vi "_get Session Name for PN.vi"(8 "error in (no error)":errorcluster, 11 "OBJ - Session in":refnum<class "Session - Root.lvclass">) -> (0 "error out":errorcluster, 2 "Session Name":string, 3 "OBJ - Session out":refnum<class "Session - Root.lvclass">)   [LabVIEW 2015, in "Session - Root.lvclass"]
doc: "Wrapped Call to maintain reverse compatibility\nOnly difference is connector pane"
uses:
  Session - Root.lvclass
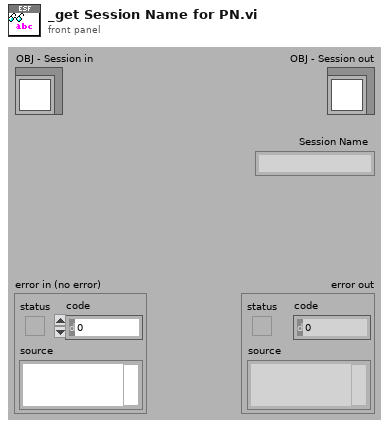
[diagram p1: front panel]
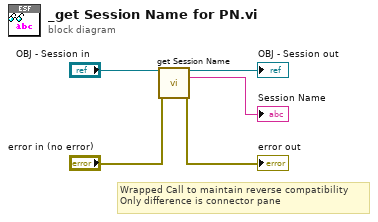
[diagram p0: block diagram]
diagram:
  # "Wrapped Call to maintain reverse compatibility\nOnly difference is connector pane"
  n1 = call "get Session Name.vi"("OBJ - Session in"="OBJ - Session in", "error in (no error)"="error in (no error)") -> ("OBJ - Session out"=→"OBJ - Session out":refnum<class "Session - Root.lvclass">, "Session Name"=→"Session Name":string, "error out"=→"error out":errorcluster)  [unwired: 11 in]
